vi "AR Drone - Gamepad NavData Video.vi"() -> ()   [LabVIEW 2015]
doc: "Example demonstrating how to control the AR Drone with a joystick or gamepad and simultaneously receive navigation and video data."
uses:
  <vilib>/LVH/AR Drone Toolkit/Decode NavData/Typedefs/NavData Demo.ctl
  <vilib>/LVH/AR Drone Toolkit/Type Defs/Flight Animations.ctl
  <vilib>/Utility/inputDevices.llb/closeJoystick.vi
  <vilib>/LVH/AR Drone Toolkit/AR Drone.lvlib
panel:
  out "Pitching speed":dbl
  out "Hover?":bool
  out "Yawing speed":sgl
  out "Vertical speed":sgl
  in  "Autopilot":bool
  in  "Stop FSM":bool
  in  "Reset":bool
  in  "Start":bool
  in  "Desired yaw":i16
  in  "Restart":bool
  in  "State":i8=1 min=1 max=33 step=1
  out "Downward loop":i8
  out "Snake loop":i8
  out "Upward loop":i8
  out "Current yaw":sgl
  out "Height":i16
  in  "Yaw speed":sgl(slide) min=-1 max=1 scale=-1.0..1.0
  in  "V speed":sgl(slide) min=-1 max=1 scale=-1.0..1.0
  in  "Pitch":sgl(slide) min=-1 max=1 scale=-1.0..1.0
  in  "Roll":sgl(slide) min=-1 max=1 scale=-1.0..1.0
  in  "display/gamepad":bool
  out "Gamepad Output":T1
  in  "Flight Animations":T2 items=["PHI_M30_DEG", "PHI_30_DEG", "THETA_M30_DEG", "THETA_30_DEG", "THETA_20DEG_YAW_200DEG", "THETA_20DEG_YAW_M2000DEG", "TURNAROUND", "TURNAROUND_GODOWN", "YAW_SHAKE", "YAW_DANCE", "PHI_DANCE", "THETA_DANCE", "VZ_DANCE", "WAVE", "PHI_THETA_MIXED", "DOUBLE_PHI_THETA_MIXED", "FLIP_AHEAD", "FLIP_BEHIND", "FLIP_LEFT", "FLIP_RIGHT", "NB_ANIM_MAYDAY"]
  out "Video Stream":picture
  out "NavData Out":T3
  out "Battery Remaining":dbl(slide) scale=0.0..100.0
  out "Axes Output":T4 {"Vertical Speed" scale=-1.0..1.0; "Yaw Speed" scale=-1.0..1.0; "Pitch" scale=-1.0..1.0; "Roll" scale=-1.0..1.0}
  in  "stop":bool
  # "Xbox Controller:\nLeft stick L/R - Roll\nLeft stick D/U - Pitch\nL/R Triggers - Vertical Speed\nRight stick L/R - Yaw Speed"
  # "Xbox Controller:\nA - take off\nB - emergency\nX - hover\nStart - Stop"
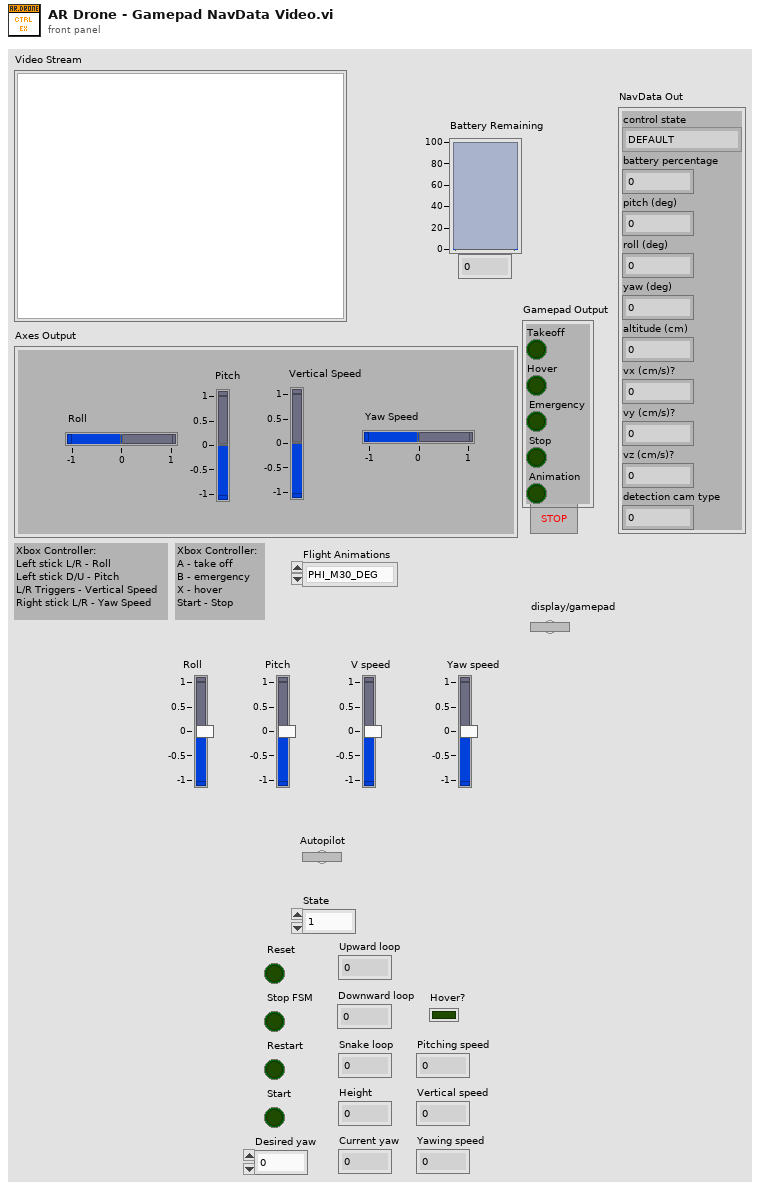
[diagram p1: front panel]
types:
  T1 = cluster{"Takeoff":bool, "Hover":bool, "Emergency":bool, "Stop":bool, "Animation":bool}
  T2 = typedef "AR Drone.lvlib/Flight Animations.ctl" = u16
  T3 = typedef "AR Drone.lvlib/NavData Demo.ctl" = cluster{"control state":enum32{"DEFAULT", "INIT", "LANDING", "FLYING", "HOVERING", "TEST", "TRANS_TAKEOFF", "TRANS_GOTOFIX", "TRANS_LANDING"}, "battery percentage":u32, "pitch (deg)":sgl, "roll (deg)":sgl, "yaw (deg)":sgl, "altitude (cm)":u32, "vx (cm/s)?":sgl, "vy (cm/s)?":sgl, "vz (cm/s)?":sgl, "detection cam type":u32}
  T4 = cluster{"Roll":dbl, "Pitch":dbl, "Vertical Speed":dbl, "Yaw Speed":dbl}
  T5 = typedef "AR Drone.lvlib/AR Drone Resource.ctl" = cluster{"UDP Control Connection":refnum<k16>, "UDP NavData Connection":refnum<k16>, "UDP Video Connection (Drone 1.0)":refnum<k16>, "TCP Video Connection (Drone 2.0)":refnum<k5>, "TCP Control Port Connection":refnum<k5>, "Drone IP address":string, "Drone Command Port":u16, "Drone NavData Port":u16, "Drone Vid Stream Port":u16, "Drone TCP Control Port":u16, "Home IP address":string, "Home Command Port":u16, "Home NavData Port":u16, "Home Vid Stream Port":u16, "Drone Version":i32}
  T6 = cluster{"Roll":sgl, "Pitch":sgl, "V speed":sgl, "Yaw speed":sgl}
  T7 = cluster{"Roll":sgl, "Pitch":sgl, "Vertical Speed":sgl, "Yaw Speed":sgl}
  T8 = cluster{"Yawing speed":sgl, "Pitching speed":dbl, "Vertical speed":sgl, "Yawing speed":sgl}
  T9 = cluster{"Roll":sgl, "Pitching speed":dbl, "V speed":sgl, "Yaw speed":sgl}
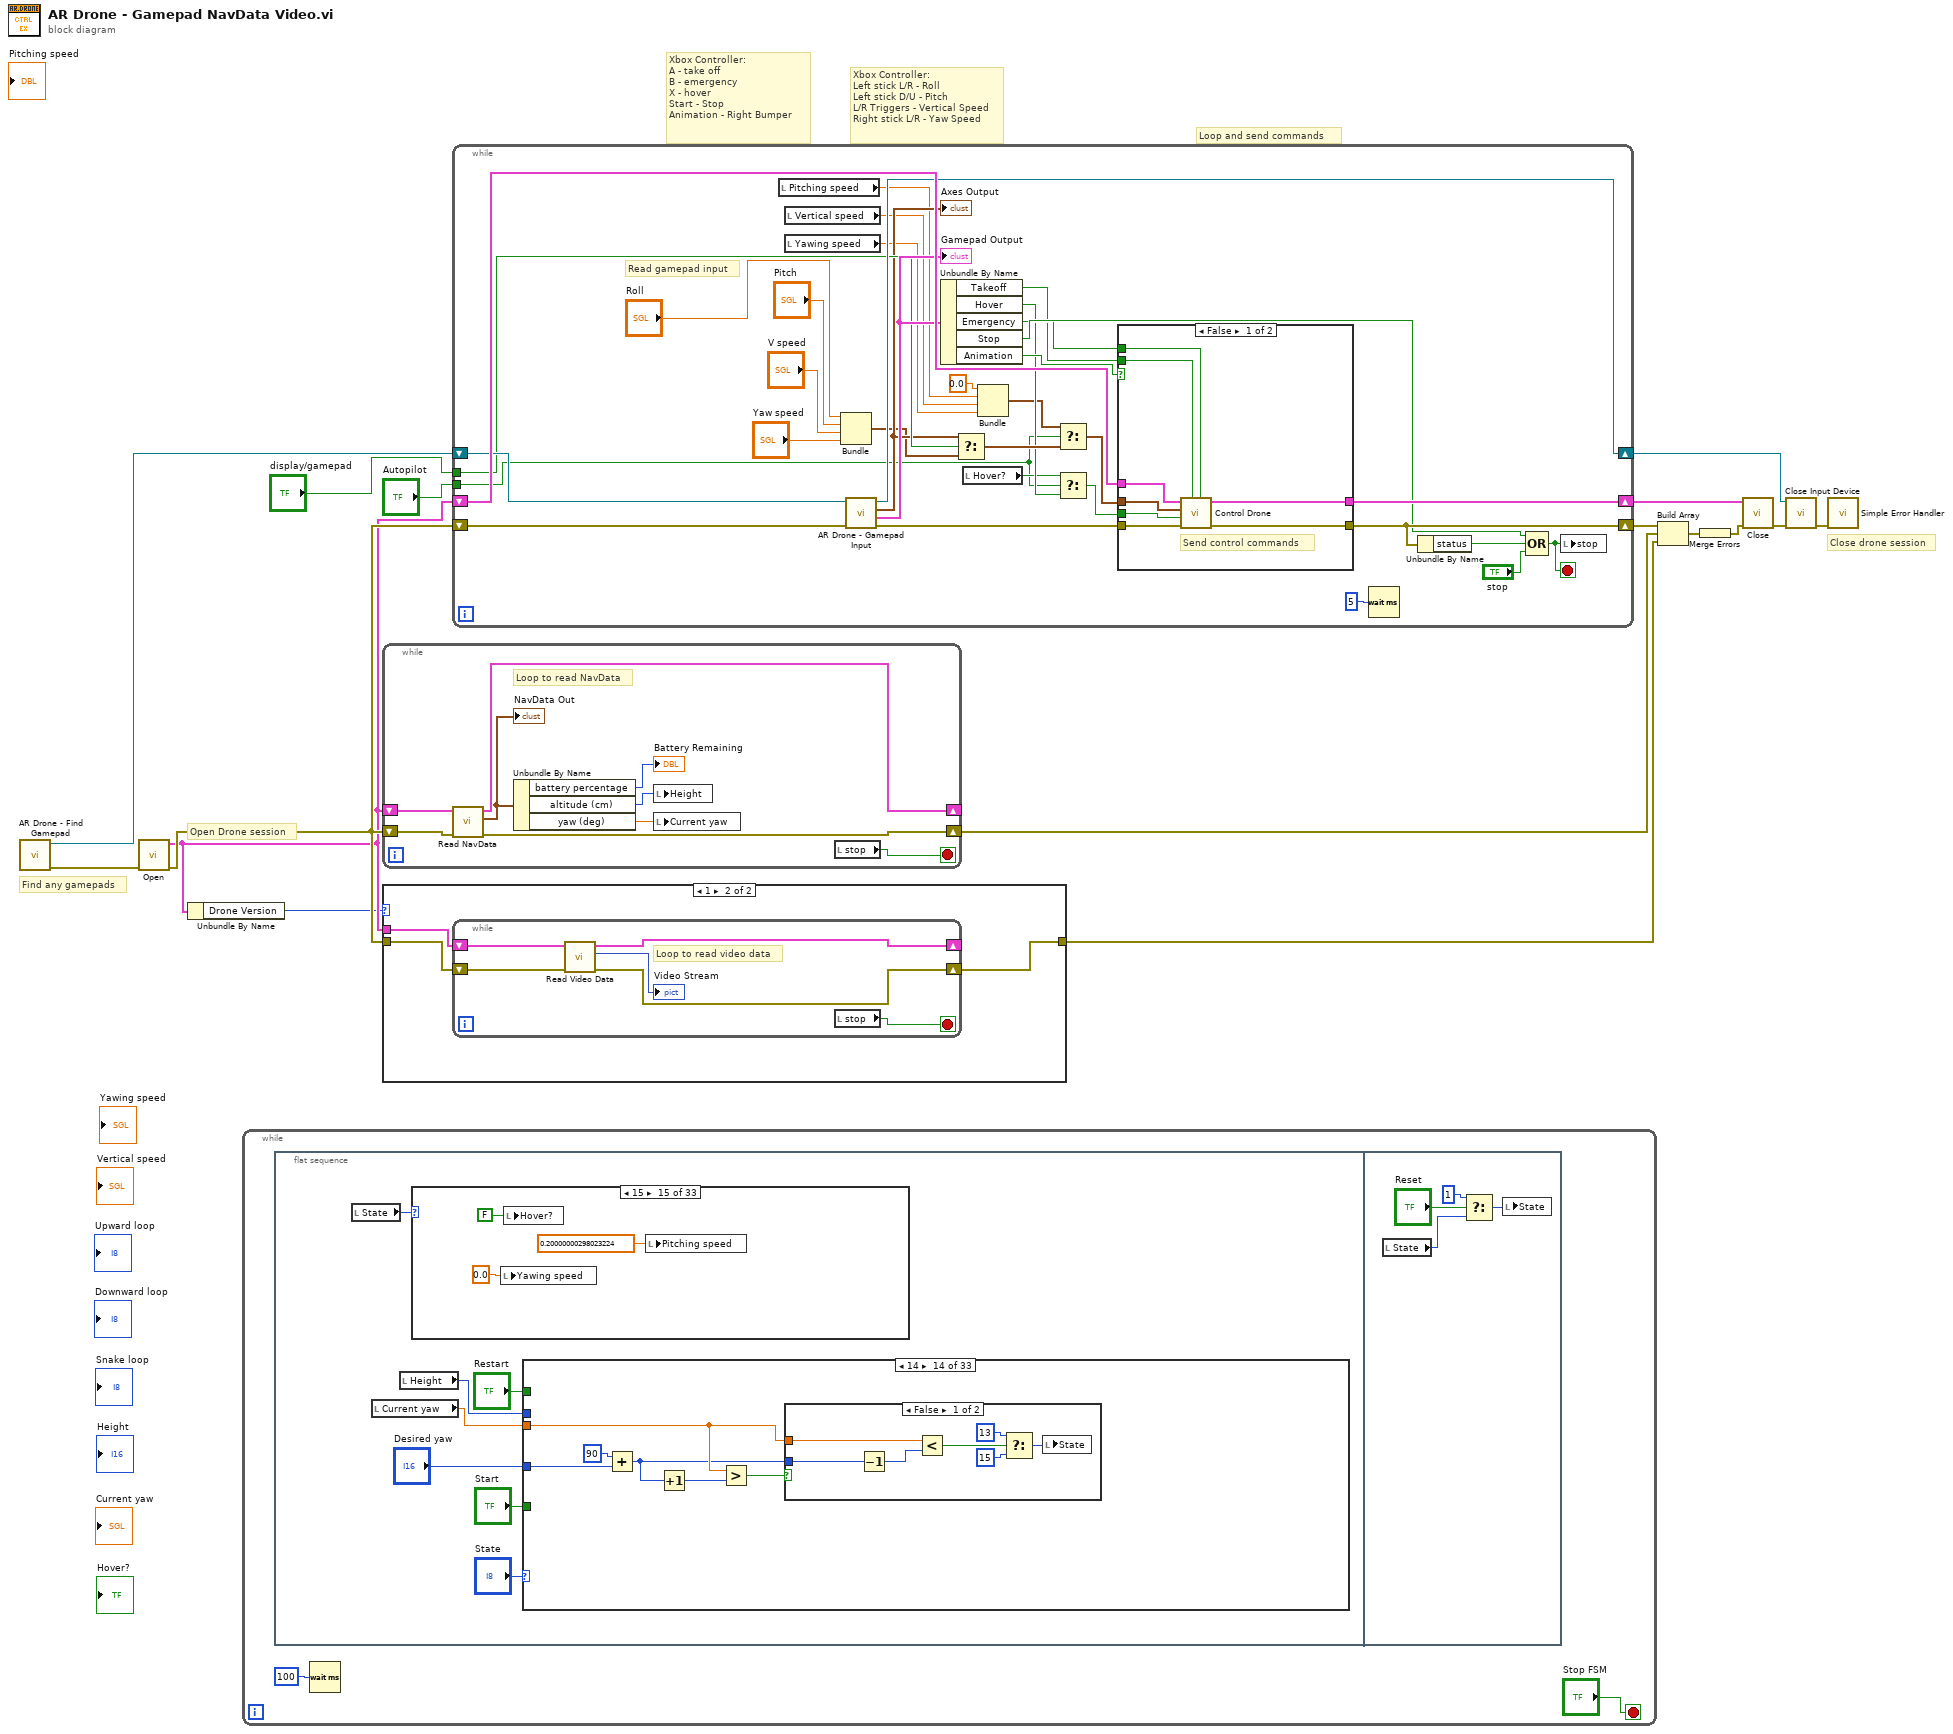
[diagram p0: block diagram]
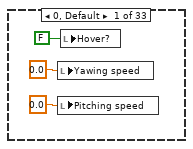
[diagram p2: hidden frame]
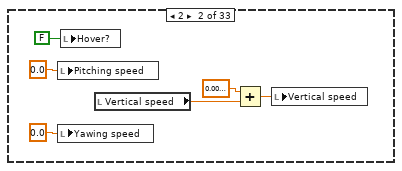
[diagram p3: hidden frame]
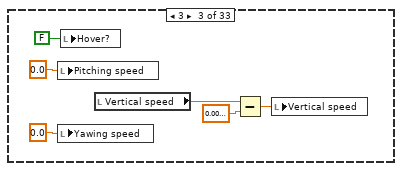
[diagram p4: hidden frame]
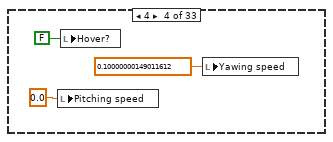
[diagram p5: hidden frame]
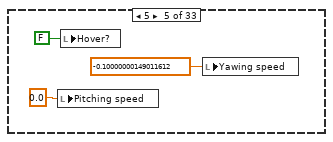
[diagram p6: hidden frame]
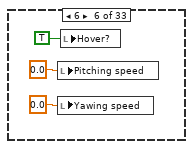
[diagram p7: hidden frame]
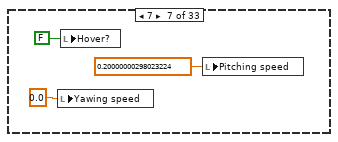
[diagram p8: hidden frame]
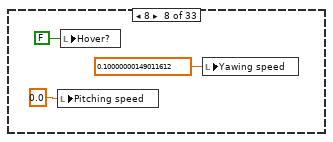
[diagram p9: hidden frame]
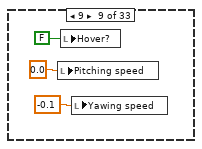
[diagram p10: hidden frame]
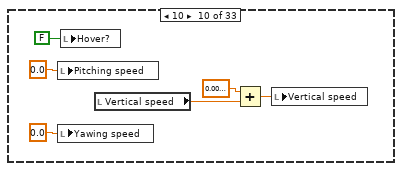
[diagram p11: hidden frame]
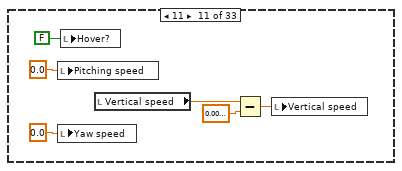
[diagram p12: hidden frame]
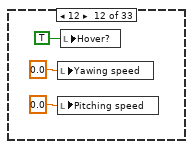
[diagram p13: hidden frame]
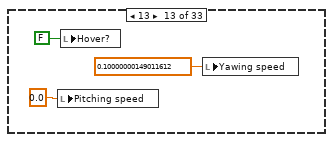
[diagram p14: hidden frame]
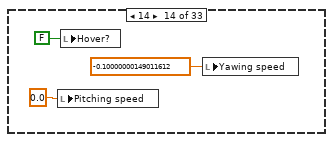
[diagram p15: hidden frame]
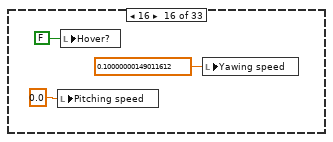
[diagram p16: hidden frame]
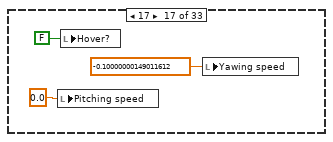
[diagram p17: hidden frame]
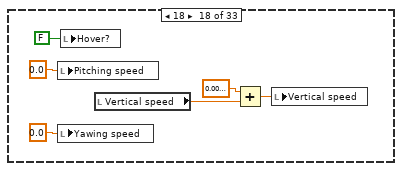
[diagram p18: hidden frame]
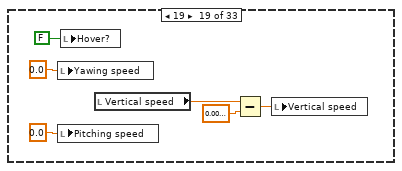
[diagram p19: hidden frame]
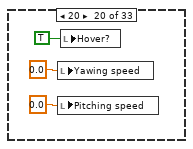
[diagram p20: hidden frame]
diagram:
  # "Loop and send commands"
  # "Close drone session"
  # "Open Drone session"
  # "Find any gamepads"
  # "Xbox Controller:\nLeft stick L/R - Roll\nLeft stick D/U - Pitch\nL/R Triggers - Vertical Speed\nRight stick L/R - Yaw Speed"
  # "Xbox Controller:\nA - take off\nB - emergency\nX - hover\nStart - Stop\nAnimation - Right Bumper"
  n1 = call "AR Drone - Find Gamepad.vi"() -> ("error out"=w11:errorcluster, "Refnum out"=w12:refnum<k1>)  [unwired: 10 in]
  n2 = call <vilib>:"Open.vi"("error in (no error)"=w11) -> ("error out"=w6:errorcluster, "AR Drone Resource"=w4:T5)  [unwired: 9 in]
  n3 = Unbundle By Name(w4) -> ("Drone Version"=w3:i32)
  n4 = while {
    stop <- "Stop FSM" stop-if-true
    n5 = flat-sequence {
      frame #0 {
        n6 = local read "State"() -> (w20:i8)
        n7 = local read "Current yaw"() -> (w23:sgl)
        n8 = local read "Height"() -> (w24:i16)
        n9 = case shown="15" w20 {
          frame 0, Default {
            n10 = local write "Yawing speed"(sgl 0.0 ("Yawing speed")) -> ()
            n11 = local write "Pitching speed"(sgl 0.0 ("Yawing speed")) -> ()
            n12 = local write "Hover?"(FALSE) -> ()
          }
          frame 2 {
            n13 = local write "Pitching speed"(sgl 0.0 ("Yawing speed")) -> ()
            n14 = local write "Yawing speed"(sgl 0.0 ("Yawing speed")) -> ()
            n15 = local write "Hover?"(FALSE) -> ()
            n16 = local read "Vertical speed"() -> (w33:sgl)
            n17 = Add(x=sgl 0.01, y=w33) -> (x+y=w34:sgl)
            n18 = local write "Vertical speed"(w34) -> ()
          }
          frame 3 {
            n19 = local write "Pitching speed"(sgl 0.0 ("Yawing speed")) -> ()
            n20 = local write "Yawing speed"(sgl 0.0 ("Yawing speed")) -> ()
            n21 = local write "Hover?"(FALSE) -> ()
            n22 = local read "Vertical speed"() -> (w39:sgl)
            n23 = Subtract(x=w39, y=sgl 0.01 ("x")) -> (x-y=w40:sgl)
            n24 = local write "Vertical speed"(w40) -> ()
          }
          frame 4 {
            n25 = local write "Pitching speed"(sgl 0.0 ("Yawing speed")) -> ()
            n26 = local write "Hover?"(FALSE) -> ()
            n27 = local write "Yawing speed"(sgl 0.1 ("Yawing speed")) -> ()
          }
          frame 5 {
            n28 = local write "Pitching speed"(sgl 0.0 ("Yawing speed")) -> ()
            n29 = local write "Hover?"(FALSE) -> ()
            n30 = local write "Yawing speed"(sgl -0.1 ("Yawing speed")) -> ()
          }
          frame 6 {
            n31 = local write "Pitching speed"(sgl 0.0 ("Yawing speed")) -> ()
            n32 = local write "Yawing speed"(sgl 0.0 ("Yawing speed")) -> ()
            n33 = local write "Hover?"(TRUE) -> ()
          }
          frame 7 {
            n34 = local write "Yawing speed"(sgl 0.0 ("Yawing speed")) -> ()
            n35 = local write "Hover?"(FALSE) -> ()
            n36 = local write "Pitching speed"(sgl 0.2 ("Yawing speed")) -> ()
          }
          frame 8 {
            n37 = local write "Pitching speed"(sgl 0.0 ("Yawing speed")) -> ()
            n38 = local write "Hover?"(FALSE) -> ()
            n39 = local write "Yawing speed"(sgl 0.1 ("Yawing speed")) -> ()
          }
          frame 9 {
            n40 = local write "Pitching speed"(sgl 0.0 ("Yawing speed")) -> ()
            n41 = local write "Hover?"(FALSE) -> ()
            n42 = local write "Yawing speed"(-0.1 ("Yawing speed")) -> ()
          }
          frame 10 {
            n43 = local write "Pitching speed"(sgl 0.0 ("Yawing speed")) -> ()
            n44 = local write "Yawing speed"(sgl 0.0 ("Yawing speed")) -> ()
            n45 = local write "Hover?"(FALSE) -> ()
            n46 = local read "Vertical speed"() -> (w64:sgl)
            n47 = Add(x=sgl 0.01, y=w64) -> (x+y=w63:sgl)
            n48 = local write "Vertical speed"(w63) -> ()
          }
          frame 11 {
            n49 = local write "Pitching speed"(sgl 0.0 ("Yawing speed")) -> ()
            n50 = local write "Yaw speed"(sgl 0.0 ("Yawing speed")) -> ()
            n51 = local write "Hover?"(FALSE) -> ()
            n52 = local read "Vertical speed"() -> (w69:sgl)
            n53 = Subtract(x=w69, y=sgl 0.01) -> (x-y=w70:sgl)
            n54 = local write "Vertical speed"(w70) -> ()
          }
          frame 12 {
            n55 = local write "Yawing speed"(sgl 0.0 ("Yawing speed")) -> ()
            n56 = local write "Pitching speed"(sgl 0.0 ("Yawing speed")) -> ()
            n57 = local write "Hover?"(TRUE) -> ()
          }
          frame 13 {
            n58 = local write "Pitching speed"(sgl 0.0 ("Yawing speed")) -> ()
            n59 = local write "Hover?"(FALSE) -> ()
            n60 = local write "Yawing speed"(sgl 0.1 ("Yawing speed")) -> ()
          }
          frame 14 {
            n61 = local write "Pitching speed"(sgl 0.0 ("Yawing speed")) -> ()
            n62 = local write "Hover?"(FALSE) -> ()
            n63 = local write "Yawing speed"(sgl -0.1 ("Yawing speed")) -> ()
          }
          frame 15 {
            n64 = local write "Yawing speed"(sgl 0.0 ("Yawing speed")) -> ()
            n65 = local write "Hover?"(FALSE) -> ()
            n66 = local write "Pitching speed"(sgl 0.2 ("Yawing speed")) -> ()
          }
          frame 16 {
            n67 = local write "Pitching speed"(sgl 0.0 ("Yawing speed")) -> ()
            n68 = local write "Hover?"(FALSE) -> ()
            n69 = local write "Yawing speed"(sgl 0.1 ("Yawing speed")) -> ()
          }
          frame 17 {
            n70 = local write "Pitching speed"(sgl 0.0 ("Yawing speed")) -> ()
            n71 = local write "Hover?"(FALSE) -> ()
            n72 = local write "Yawing speed"(sgl -0.1 ("Yawing speed")) -> ()
          }
          frame 18 {
            n73 = local write "Pitching speed"(sgl 0.0 ("Yawing speed")) -> ()
            n74 = local write "Yawing speed"(sgl 0.0 ("Yawing speed")) -> ()
            n75 = local write "Hover?"(FALSE) -> ()
            n76 = local read "Vertical speed"() -> (w94:sgl)
            n77 = Add(x=sgl 0.01, y=w94) -> (x+y=w93:sgl)
            n78 = local write "Vertical speed"(w93) -> ()
          }
          frame 19 {
            n79 = local write "Yawing speed"(sgl 0.0 ("Yawing speed")) -> ()
            n80 = local write "Pitching speed"(sgl 0.0 ("Yawing speed")) -> ()
            n81 = local write "Hover?"(FALSE) -> ()
            n82 = local read "Vertical speed"() -> (w99:sgl)
            n83 = Subtract(x=w99, y=sgl 0.01) -> (x-y=w100:sgl)
            n84 = local write "Vertical speed"(w100) -> ()
          }
          frame 20 {
            n85 = local write "Yawing speed"(sgl 0.0 ("Yawing speed")) -> ()
            n86 = local write "Pitching speed"(sgl 0.0 ("Yawing speed")) -> ()
            n87 = local write "Hover?"(TRUE) -> ()
          }
          frame 21 {
            n88 = local write "Yawing speed"(sgl 0.0 ("Yawing speed")) -> ()
            n89 = local write "Pitching speed"(sgl 0.0 ("Yawing speed")) -> ()
            n90 = local write "Hover?"(FALSE) -> ()
          }
          frame 22 {
            n91 = local write "Pitching speed"(sgl 0.0 ("Yawing speed")) -> ()
            n92 = local write "Hover?"(FALSE) -> ()
            n93 = local write "Yawing speed"(sgl 0.1 ("Yawing speed")) -> ()
          }
          frame 23 {
            n94 = local write "Pitching speed"(sgl 0.0 ("Yawing speed")) -> ()
            n95 = local write "Hover?"(FALSE) -> ()
            n96 = local write "Yawing speed"(sgl -0.1 ("Yawing speed")) -> ()
          }
          frame 24 {
            n97 = local write "Yawing speed"(sgl 0.0 ("Yawing speed")) -> ()
            n98 = local write "Pitching speed"(sgl 0.0 ("Yawing speed")) -> ()
            n99 = local write "Hover?"(FALSE) -> ()
            n100 = local read "Vertical speed"() -> (w118:sgl)
            n101 = Add(x=sgl 0.01, y=w118) -> (x+y=w117:sgl)
            n102 = local write "Vertical speed"(w117) -> ()
          }
          frame 25 {
            n103 = local write "Pitching speed"(sgl 0.0 ("Yawing speed")) -> ()
            n104 = local write "Yawing speed"(sgl 0.0 ("Yawing speed")) -> ()
            n105 = local write "Hover?"(FALSE) -> ()
            n106 = local read "Vertical speed"() -> (w123:sgl)
            n107 = Subtract(x=w123, y=sgl 0.01) -> (x-y=w124:sgl)
            n108 = local write "Vertical speed"(w124) -> ()
          }
          frame 26 {
            n109 = local write "Yawing speed"(sgl 0.0 ("Yawing speed")) -> ()
            n110 = local write "Pitching speed"(sgl 0.0 ("Yawing speed")) -> ()
            n111 = local write "Hover?"(TRUE) -> ()
          }
          frame 27 {
            n112 = local write "Pitching speed"(sgl 0.0 ("Yawing speed")) -> ()
            n113 = local write "Hover?"(FALSE) -> ()
            n114 = local write "Yawing speed"(sgl 0.1 ("Yawing speed")) -> ()
          }
          frame 28 {
            n115 = local write "Pitching speed"(sgl 0.0 ("Yawing speed")) -> ()
            n116 = local write "Hover?"(FALSE) -> ()
            n117 = local write "Yawing speed"(sgl -0.1 ("Yawing speed")) -> ()
          }
          frame 29 {
            n118 = local write "Yawing speed"(sgl 0.0 ("Yawing speed")) -> ()
            n119 = local write "Hover?"(FALSE) -> ()
            n120 = local write "Pitching speed"(sgl 0.2 ("Yawing speed")) -> ()
          }
          frame 30 {
            n121 = local write "Pitching speed"(sgl 0.0 ("Yawing speed")) -> ()
            n122 = local write "Hover?"(FALSE) -> ()
            n123 = local write "Yawing speed"(sgl 0.1 ("Yawing speed")) -> ()
          }
          frame 31 {
            n124 = local write "Pitching speed"(sgl 0.0 ("Yawing speed")) -> ()
            n125 = local write "Hover?"(FALSE) -> ()
            n126 = local write "Yawing speed"(sgl -0.1 ("Yawing speed")) -> ()
          }
          frame 32 {
            n127 = local write "Yawing speed"(sgl 0.0 ("Yawing speed")) -> ()
            n128 = local write "Pitching speed"(sgl 0.0 ("Yawing speed")) -> ()
            n129 = local write "Hover?"(TRUE) -> ()
          }
          frame 33 {
            n130 = local write "Yawing speed"(sgl 0.0 ("Yawing speed")) -> ()
            n131 = local write "Pitching speed"(sgl 0.0 ("Yawing speed")) -> ()
            n132 = local write "Hover?"(FALSE) -> ()
          }
        }
        n133 = case shown="14" "State" {
          tunnel: "Start" -> [w152 _ _ _ _ _ _ _ _ _ _ _ _ _ _ _ _ _ _ _ _ _ _ _ _ _ _ _ _ _ _ _ _]
          tunnel: w24 -> [_ w156 w166 _ _ _ _ _ _ w226 w236 _ _ _ _ _ _ w309 w319 _ _ _ _ w359 w369 _ _ _ _ _ _ _ _]
          tunnel: w23 -> [_ _ _ w178 w189 _ _ w203 w215 _ _ _ w255 w269 _ w281 w295 _ _ _ _ w331 w345 _ _ _ w385 w399 _ w415 w429 _ _]
          tunnel: "Desired yaw" -> [_ _ _ w176 w188 _ _ w202 w214 _ _ _ w252 w268 _ w282 w296 _ _ _ _ w332 w346 _ _ _ w386 w400 _ w414 w428 _ _]
          tunnel: "Restart" -> [_ _ _ _ _ _ _ _ _ _ _ _ _ _ _ _ _ _ _ _ _ _ _ _ _ _ _ _ _ _ _ _ w453]
          frame Default {
            n134 = Select(t=i8 2, s=w152, f=i8 1) -> (s? t:f=w155:i8)
            n135 = local write "Upward loop"(i8 5 ("pic loop")) -> ()
            n136 = local write "Downward loop"(i8 5 ("pic loop 2")) -> ()
            n137 = local write "Snake loop"(i8 3 ("snake loop")) -> ()
            n138 = local write "State"(w155) -> ()
          }
          frame 2 {
            n139 = Greater?(x=w156, y=i16 152) -> (0:w157:bool)
            n140 = case shown="False" w157 {
              tunnel: w156 -> [w164 _]
              frame False {
                n141 = Less?(x=w164, y=i16 148) -> (x < y?=w162:bool)
                n142 = Select(t=i8 2, s=w162, f=i8 4) -> (s? t:f=w159:i8)
                n143 = local write "State"(w159) -> ()
              }
              frame True {
                n144 = local write "State"(i8 3 ("state")) -> ()
              }
            }
          }
          frame 3 {
            n145 = Greater?(x=w166, y=i16 152) -> (0:w168:bool)
            n146 = case shown="True" w168 {
              tunnel: w166 -> [w174 _]
              frame False {
                n147 = Less?(x=w174, y=i16 148) -> (x < y?=w172:bool)
                n148 = Select(t=i8 2, s=w172, f=i8 4) -> (s? t:f=w169:i8)
                n149 = local write "State"(w169) -> ()
              }
              frame True {
                n150 = local write "State"(i8 3 ("state")) -> ()
              }
            }
          }
          frame 4 {
            n151 = Increment(x=w176) -> (x+1=w177:i16)
            n152 = Greater?(x=w178, y=w177) -> (0:w179:bool)
            n153 = case shown="True" w179 {
              tunnel: w178 -> [w186 _]
              tunnel: w176 -> [w180 _]
              frame False {
                n154 = Decrement(x=w180) -> (x-1=w181:i16)
                n155 = Less?(x=w186, y=w181) -> (x < y?=w185:bool)
                n156 = Select(t=i8 4, s=w185, f=i8 6) -> (s? t:f=w182:i8)
                n157 = local write "State"(w182) -> ()
              }
              frame True {
                n158 = local write "State"(i8 5 ("state")) -> ()
              }
            }
          }
          frame 5 {
            n159 = Increment(x=w188) -> (x+1=w191:i16)
            n160 = Greater?(x=w189, y=w191) -> (0:w190:bool)
            n161 = case shown="False" w190 {
              tunnel: w189 -> [w198 _]
              tunnel: w188 -> [w192 _]
              frame False {
                n162 = Decrement(x=w192) -> (x-1=w193:i16)
                n163 = Less?(x=w198, y=w193) -> (x < y?=w197:bool)
                n164 = Select(t=i8 4, s=w197, f=i8 6) -> (s? t:f=w194:i8)
                n165 = local write "State"(w194) -> ()
              }
              frame True {
                n166 = local write "State"(i8 5 ("state")) -> ()
              }
            }
          }
          frame 6 {
            n167 = flat-sequence {
              frame #0 {
                n168 = call "Time Delay"() -> ()  [unwired: 11 in, 1 out]
              }
              frame #1 {
                n169 = local write "State"(i8 7 ("state")) -> ()
              }
            }
          }
          frame 7 {
            n170 = flat-sequence {
              frame #0 {
                n171 = call "Time Delay2"() -> ()  [unwired: 11 in, 1 out]
              }
              frame #1 {
                n172 = local write "State"(i8 8 ("state")) -> ()
              }
            }
          }
          frame 8 {
            n173 = Increment(x=w202) -> (x+1=w204:i16)
            n174 = Greater?(x=w203, y=w204) -> (0:w205:bool)
            n175 = case shown="False" w205 {
              tunnel: w203 -> [w212 _]
              tunnel: w202 -> [w206 _]
              frame False {
                n176 = Decrement(x=w206) -> (x-1=w207:i16)
                n177 = Less?(x=w212, y=w207) -> (x < y?=w211:bool)
                n178 = Select(t=i8 8, s=w211, f=i8 10) -> (s? t:f=w208:i8)
                n179 = local write "State"(w208) -> ()
              }
              frame True {
                n180 = local write "State"(i8 9 ("state")) -> ()
              }
            }
          }
          frame 9 {
            n181 = Increment(x=w214) -> (x+1=w217:i16)
            n182 = Greater?(x=w215, y=w217) -> (0:w216:bool)
            n183 = case shown="True" w216 {
              tunnel: w215 -> [w224 _]
              tunnel: w214 -> [w218 _]
              frame False {
                n184 = Decrement(x=w218) -> (x-1=w219:i16)
                n185 = Less?(x=w224, y=w219) -> (x < y?=w223:bool)
                n186 = Select(t=i8 8, s=w223, f=i8 10) -> (s? t:f=w220:i8)
                n187 = local write "State"(w220) -> ()
              }
              frame True {
                n188 = local write "State"(i8 9 ("state")) -> ()
              }
            }
          }
          frame 10 {
            n189 = Greater?(x=w226, y=i16 152) -> (0:w227:bool)
            n190 = case shown="False" w227 {
              tunnel: w226 -> [w234 _]
              frame False {
                n191 = Less?(x=w234, y=i16 148) -> (x < y?=w232:bool)
                n192 = Select(t=i8 10, s=w232, f=i8 12) -> (s? t:f=w229:i8)
                n193 = local write "State"(w229) -> ()
              }
              frame True {
                n194 = local write "State"(i8 11 ("state")) -> ()
              }
            }
          }
          frame 11 {
            n195 = Greater?(x=w236, y=i16 152) -> (0:w238:bool)
            n196 = case shown="False" w238 {
              tunnel: w236 -> [w244 _]
              frame False {
                n197 = Less?(x=w244, y=i16 148) -> (x < y?=w242:bool)
                n198 = Select(t=i8 10, s=w242, f=i8 12) -> (s? t:f=w239:i8)
                n199 = local write "State"(w239) -> ()
              }
              frame True {
                n200 = local write "State"(i8 11 ("state")) -> ()
              }
            }
          }
          frame 12 {
            n201 = flat-sequence {
              frame #0 {
                n202 = call "Time Delay3"() -> ()  [unwired: 11 in, 1 out]
              }
              frame #1 {
                n203 = local read "Upward loop"() -> (w250:i8)
                n204 = Decrement(x=w250) -> (x-1=w251:i8)
                n205 = local write "Upward loop"(w251) -> ()
                n206 = Equal To 0?(x=w251) -> (x = 0?=w246:bool)
                n207 = Select(t=i8 13, s=w246, f=i8 7) -> (s? t:f=w249:i8)
                n208 = local write "State"(w249) -> ()
              }
            }
          }
          frame 13 {
            n209 = Add(x=i16 90, y=w252) -> (x+y=w253:i16)
            n210 = Increment(x=w253) -> (x+1=w257:i16)
            n211 = Greater?(x=w255, y=w257) -> (0:w256:bool)
            n212 = case shown="True" w256 {
              tunnel: w255 -> [w264 _]
              tunnel: w253 -> [w258 _]
              frame False {
                n213 = Decrement(x=w258) -> (x-1=w259:i16)
                n214 = Less?(x=w264, y=w259) -> (x < y?=w263:bool)
                n215 = Select(t=i8 13, s=w263, f=i8 15) -> (s? t:f=w260:i8)
                n216 = local write "State"(w260) -> ()
              }
              frame True {
                n217 = local write "State"(i8 14 ("state")) -> ()
              }
            }
          }
          frame 14 {
            n218 = Add(x=i16 90, y=w268) -> (x+y=w267:i16)
            n219 = Increment(x=w267) -> (x+1=w270:i16)
            n220 = Greater?(x=w269, y=w270) -> (0:w271:bool)
            n221 = case shown="False" w271 {
              tunnel: w269 -> [w278 _]
              tunnel: w267 -> [w272 _]
              frame False {
                n222 = Decrement(x=w272) -> (x-1=w273:i16)
                n223 = Less?(x=w278, y=w273) -> (x < y?=w277:bool)
                n224 = Select(t=i8 13, s=w277, f=i8 15) -> (s? t:f=w274:i8)
                n225 = local write "State"(w274) -> ()
              }
              frame True {
                n226 = local write "State"(i8 14 ("state")) -> ()
              }
            }
          }
          frame 15 {
            n227 = flat-sequence {
              frame #0 {
                n228 = call "Time Delay4"() -> ()  [unwired: 11 in, 1 out]
              }
              frame #1 {
                n229 = local write "State"(i8 16 ("state")) -> ()
              }
            }
          }
          frame 16 {
            n230 = Add(x=i16 180, y=w282) -> (x+y=w286:i16)
            n231 = Increment(x=w286) -> (x+1=w283:i16)
            n232 = Greater?(x=w281, y=w283) -> (0:w284:bool)
            n233 = case shown="True" w284 {
              tunnel: w281 -> [w293 _]
              tunnel: w286 -> [w287 _]
              frame False {
                n234 = Decrement(x=w287) -> (x-1=w288:i16)
                n235 = Less?(x=w293, y=w288) -> (x < y?=w292:bool)
                n236 = Select(t=i8 16, s=w292, f=i8 18) -> (s? t:f=w289:i8)
                n237 = local write "State"(w289) -> ()
              }
              frame True {
                n238 = local write "State"(i8 17 ("state")) -> ()
              }
            }
          }
          frame 17 {
            n239 = Add(x=i16 180, y=w296) -> (x+y=w300:i16)
            n240 = Increment(x=w300) -> (x+1=w297:i16)
            n241 = Greater?(x=w295, y=w297) -> (0:w298:bool)
            n242 = case shown="True" w298 {
              tunnel: w295 -> [w307 _]
              tunnel: w300 -> [w301 _]
              frame False {
                n243 = Decrement(x=w301) -> (x-1=w302:i16)
                n244 = Less?(x=w307, y=w302) -> (x < y?=w306:bool)
                n245 = Select(t=i8 16, s=w306, f=i8 18) -> (s? t:f=w303:i8)
                n246 = local write "State"(w303) -> ()
              }
              frame True {
                n247 = local write "State"(i8 17 ("state")) -> ()
              }
            }
          }
          frame 18 {
            n248 = Greater?(x=w309, y=i16 152) -> (0:w311:bool)
            n249 = case shown="True" w311 {
              tunnel: w309 -> [w317 _]
              frame False {
                n250 = Less?(x=w317, y=i16 148) -> (x < y?=w315:bool)
                n251 = Select(t=i8 18, s=w315, f=i8 20) -> (s? t:f=w312:i8)
                n252 = local write "State"(w312) -> ()
              }
              frame True {
                n253 = local write "State"(i8 19 ("state")) -> ()
              }
            }
          }
          frame 19 {
            n254 = Greater?(x=w319, y=i16 152) -> (0:w321:bool)
            n255 = case shown="True" w321 {
              tunnel: w319 -> [w327 _]
              frame False {
                n256 = Less?(x=w327, y=i16 148) -> (x < y?=w325:bool)
                n257 = Select(t=i8 18, s=w325, f=i8 20) -> (s? t:f=w322:i8)
                n258 = local write "State"(w322) -> ()
              }
              frame True {
                n259 = local write "State"(i8 19 ("state")) -> ()
              }
            }
          }
          frame 20 {
            n260 = flat-sequence {
              frame #0 {
                n261 = call "Time Delay5"() -> ()  [unwired: 11 in, 1 out]
              }
              frame #1 {
                n262 = local write "State"(i8 21 ("state")) -> ()
              }
            }
          }
          frame 21 {
            n263 = flat-sequence {
              frame #0 {
                n264 = call "Time Delay6"() -> ()  [unwired: 11 in, 1 out]
              }
              frame #1 {
                n265 = local write "State"(i8 22 ("state")) -> ()
              }
            }
          }
          frame 22 {
            n266 = Add(x=i16 180, y=w332) -> (x+y=w333:i16)
            n267 = Increment(x=w333) -> (x+1=w336:i16)
            n268 = Greater?(x=w331, y=w336) -> (0:w335:bool)
            n269 = case shown="True" w335 {
              tunnel: w331 -> [w343 _]
              tunnel: w333 -> [w337 _]
              frame False {
                n270 = Decrement(x=w337) -> (x-1=w338:i16)
                n271 = Less?(x=w343, y=w338) -> (x < y?=w342:bool)
                n272 = Select(t=i8 22, s=w342, f=i8 24) -> (s? t:f=w339:i8)
                n273 = local write "State"(w339) -> ()
              }
              frame True {
                n274 = local write "State"(i8 23 ("state")) -> ()
              }
            }
          }
          frame 23 {
            n275 = Add(x=i16 180, y=w346) -> (x+y=w347:i16)
            n276 = Increment(x=w347) -> (x+1=w350:i16)
            n277 = Greater?(x=w345, y=w350) -> (0:w349:bool)
            n278 = case shown="True" w349 {
              tunnel: w345 -> [w357 _]
              tunnel: w347 -> [w351 _]
              frame False {
                n279 = Decrement(x=w351) -> (x-1=w352:i16)
                n280 = Less?(x=w357, y=w352) -> (x < y?=w356:bool)
                n281 = Select(t=i8 22, s=w356, f=i8 24) -> (s? t:f=w353:i8)
                n282 = local write "State"(w353) -> ()
              }
              frame True {
                n283 = local write "State"(i8 23 ("state")) -> ()
              }
            }
          }
          frame 24 {
            n284 = Greater?(x=w359, y=i16 152) -> (0:w360:bool)
            n285 = case shown="True" w360 {
              tunnel: w359 -> [w367 _]
              frame False {
                n286 = Less?(x=w367, y=i16 148) -> (x < y?=w365:bool)
                n287 = Select(t=i8 24, s=w365, f=i8 26) -> (s? t:f=w362:i8)
                n288 = local write "State"(w362) -> ()
              }
              frame True {
                n289 = local write "State"(i8 25 ("state")) -> ()
              }
            }
          }
          frame 25 {
            n290 = Greater?(x=w369, y=i16 152) -> (0:w370:bool)
            n291 = case shown="True" w370 {
              tunnel: w369 -> [w377 _]
              frame False {
                n292 = Less?(x=w377, y=i16 148) -> (x < y?=w375:bool)
                n293 = Select(t=i8 24, s=w375, f=i8 26) -> (s? t:f=w372:i8)
                n294 = local write "State"(w372) -> ()
              }
              frame True {
                n295 = local write "State"(i8 25 ("state")) -> ()
              }
            }
          }
          frame 26 {
            n296 = flat-sequence {
              frame #0 {
                n297 = call "Time Delay7"() -> ()  [unwired: 11 in, 1 out]
              }
              frame #1 {
                n298 = local read "Downward loop"() -> (w383:i8)
                n299 = Decrement(x=w383) -> (x-1=w384:i8)
                n300 = local write "Downward loop"(w384) -> ()
                n301 = Equal To 0?(x=w384) -> (x = 0?=w379:bool)
                n302 = Select(t=i8 27, s=w379, f=i8 21) -> (s? t:f=w382:i8)
                n303 = local write "State"(w382) -> ()
              }
            }
          }
          frame 27 {
            n304 = Add(x=i16 90, y=w386) -> (x+y=w390:i16)
            n305 = Increment(x=w390) -> (x+1=w387:i16)
            n306 = Greater?(x=w385, y=w387) -> (0:w388:bool)
            n307 = case shown="True" w388 {
              tunnel: w385 -> [w397 _]
              tunnel: w390 -> [w391 _]
              frame False {
                n308 = Decrement(x=w391) -> (x-1=w392:i16)
                n309 = Less?(x=w397, y=w392) -> (x < y?=w396:bool)
                n310 = Select(t=i8 27, s=w396, f=i8 29) -> (s? t:f=w393:i8)
                n311 = local write "State"(w393) -> ()
              }
              frame True {
                n312 = local write "State"(i8 28 ("state")) -> ()
              }
            }
          }
          frame 28 {
            n313 = Add(x=i16 90, y=w400) -> (x+y=w401:i16)
            n314 = Increment(x=w401) -> (x+1=w404:i16)
            n315 = Greater?(x=w399, y=w404) -> (0:w403:bool)
            n316 = case shown="False" w403 {
              tunnel: w399 -> [w411 _]
              tunnel: w401 -> [w405 _]
              frame False {
                n317 = Decrement(x=w405) -> (x-1=w406:i16)
                n318 = Less?(x=w411, y=w406) -> (x < y?=w410:bool)
                n319 = Select(t=i8 27, s=w410, f=i8 29) -> (s? t:f=w407:i8)
                n320 = local write "State"(w407) -> ()
              }
              frame True {
                n321 = local write "State"(i8 28 ("state")) -> ()
              }
            }
          }
          frame 29 {
            n322 = flat-sequence {
              frame #0 {
                n323 = call "Time Delay8"() -> ()  [unwired: 11 in, 1 out]
              }
              frame #1 {
                n324 = local write "State"(i8 30 ("state")) -> ()
              }
            }
          }
          frame 30 {
            n325 = Add(x=i16 180, y=w414) -> (x+y=w416:i16)
            n326 = Increment(x=w416) -> (x+1=w419:i16)
            n327 = Greater?(x=w415, y=w419) -> (0:w418:bool)
            n328 = case shown="True" w418 {
              tunnel: w415 -> [w426 _]
              tunnel: w416 -> [w420 _]
              frame False {
                n329 = Decrement(x=w420) -> (x-1=w421:i16)
                n330 = Less?(x=w426, y=w421) -> (x < y?=w425:bool)
                n331 = Select(t=i8 30, s=w425, f=i8 32) -> (s? t:f=w422:i8)
                n332 = local write "State"(w422) -> ()
              }
              frame True {
                n333 = local write "State"(i8 31 ("state")) -> ()
              }
            }
          }
          frame 31 {
            n334 = Add(x=i16 180, y=w428) -> (x+y=w430:i16)
            n335 = Increment(x=w430) -> (x+1=w433:i16)
            n336 = Greater?(x=w429, y=w433) -> (0:w432:bool)
            n337 = case shown="True" w432 {
              tunnel: w429 -> [w440 _]
              tunnel: w430 -> [w434 _]
              frame False {
                n338 = Decrement(x=w434) -> (x-1=w435:i16)
                n339 = Less?(x=w440, y=w435) -> (x < y?=w439:bool)
                n340 = Select(t=i8 30, s=w439, f=i8 32) -> (s? t:f=w436:i8)
                n341 = local write "State"(w436) -> ()
              }
              frame True {
                n342 = local write "State"(i8 31 ("state")) -> ()
              }
            }
          }
          frame 32 {
            n343 = flat-sequence {
              frame #0 {
                n344 = call "Time Delay9"() -> ()  [unwired: 11 in, 1 out]
              }
              frame #1 {
                n345 = local write "Upward loop"(i8 5 ("pic loop 1")) -> ()
                n346 = local write "Downward loop"(i8 5 ("pic loop 2")) -> ()
                n347 = local read "Snake loop"() -> (w446:i8)
                n348 = Decrement(x=w446) -> (x-1=w447:i8)
                n349 = Equal To 0?(x=w447) -> (x = 0?=w442:bool)
                n350 = local write "Snake loop"(w447) -> ()
                n351 = Select(t=i8 33, s=w442, f=i8 7) -> (s? t:f=w445:i8)
                n352 = local write "State"(w445) -> ()
              }
            }
          }
          frame 33 {
            n353 = Select(t=i8 1, s=w453, f=i8 33) -> (s? t:f=w452:i8)
            n354 = local write "State"(w452) -> ()
          }
        }
      }
      frame #1 {
        n355 = local read "State"() -> (w456:i8)
        n356 = Select(t=i8 1, s="Reset", f=w456) -> (s? t:f=w457:i8)
        n357 = local write "State"(w457) -> ()
      }
    }
    n358 = Wait (ms)(milliseconds to wait=u32 100) -> ()  [unwired: 1 out]
  }
  n359 = while {
    shift-right: [w465] -> _
    shift-left: w4 -> [w466]
    shift-right: [w463] -> w8
    shift-left: w6 -> [w464]
    stop <- w461 stop-if-true
    # "Loop to read NavData"
    n360 = call <vilib>:"Read NavData.vi"("error in (no error)"=w464, "AR Drone Resource"=w466) -> ("error out"=w463:errorcluster, "NavData Out"=w460:T3, "AR Drone Resource Out"=w465:T5)  [unwired: 7 in]
    "NavData Out" <- w460
    n361 = Unbundle By Name(w460) -> ("battery percentage"=→"Battery Remaining":u32, "altitude (cm)"=w459:u32, "yaw (deg)"=w458:sgl)
    n362 = local write "Height"(w459) -> ()
    n363 = local write "Current yaw"(w458) -> ()
    n364 = local read "stop"() -> (w461:bool)
  }
  n365 = case shown="1" w3 {
    tunnel: w4 -> [_ w470]
    tunnel: [w467 w469] -> w7
    tunnel: w6 -> [w467 w468]
    frame 2, Default {
      # "If Drone 2.0, no streaming in line"
    }
    frame 1 {
      n366 = while {
        shift-right: [w474] -> _
        shift-left: w470 -> [w476]
        shift-right: [w473] -> w469
        shift-left: w468 -> [w475]
        stop <- w471 stop-if-true
        # "Loop to read video data"
        n367 = call <vilib>:"Read Video Data.vi"("error in (no error)"=w475, "AR Drone Resource"=w476) -> ("error out"=w473:errorcluster, "Video Stream"=→"Video Stream":picture, "AR Drone Resource Out"=w474:T5)  [unwired: 7 in]
        n368 = local read "stop"() -> (w471:bool)
      }
    }
  }
  n369 = while {
    shift-right: [w509] -> w16
    shift-left: w4 -> [w510]
    shift-right: [w508] -> w9
    shift-left: w6 -> [w503]
    shift-right: [w500] -> w15
    shift-left: w12 -> [w504]
    tunnel: "display/gamepad" -> [w494]
    tunnel: "Autopilot" -> [w482]
    stop <- w496 stop-if-true
    # "Read gamepad input"
    n370 = local read "Pitching speed"() -> (w481:dbl)
    n371 = local read "Vertical speed"() -> (w478:sgl)
    n372 = local read "Yawing speed"() -> (w479:sgl)
    n373 = Bundle("Roll"="Roll", "Pitch"="Pitch", "V speed"="V speed", "Yaw speed"="Yaw speed") -> (w489:T6)  [unwired: 1 in]
    n374 = call "AR Drone - Gamepad Input.vi"("error in (no error)"=w503, "Refnum in"=w504) -> ("error out"=w502:errorcluster, "Gamepad Output"=w501:T1, "Control Cluster"=w493:T7, "Refnum out"=w500:refnum<k1>)  [unwired: 6 in]
    "Axes Output" <- w493
    "Gamepad Output" <- w501
    n375 = Unbundle By Name(w501) -> ("Takeoff"=w497:bool, "Hover"=w484:bool, "Emergency"=w498:bool, "Stop"=w499:bool, "Animation"=w495:bool)
    n376 = Select(t=w493, s=w494, f=w489) -> (s? t:f=w487:T6)
    n377 = local read "Hover?"() -> (w483:bool)
    n378 = Bundle("Yawing speed"=sgl 0.0, "Pitching speed"=w481, "Vertical speed"=w478, "Yawing speed"=w479) -> (w477:T8)  [unwired: 1 in]
    n379 = Select(t=w477, s=w482, f=w487) -> (s? t:f=w486:T9)
    n380 = Select(t=w483, s=w482, f=w484) -> (s? t:f=w485:bool)
    n381 = case shown="False" w495 {
      tunnel: w510 -> [w518 w521]
      tunnel: [w517 w519] -> w509
      tunnel: [w516 w520] -> w508
      tunnel: w502 -> [w515 w522]
      tunnel: w486 -> [w514 _]
      tunnel: w498 -> [w513 _]
      tunnel: w485 -> [w512 _]
      tunnel: w497 -> [w511 _]
      frame False {
        # "Send control commands"
        n382 = call <vilib>:"Control Drone.vi"("Emergency Landing"=w513, "Takeoff/Land"=w511, "error in (no error)"=w515, "Hover"=w512, "Control Cluster"=w514, "AR Drone Resource"=w518) -> ("error out"=w516:errorcluster, "AR Drone Resource Out"=w517:T5)  [unwired: 4 in]
      }
      frame True {
        n383 = call <vilib>:"Execute Animation.vi"("error in (no error)"=w522, "Flight Animation"="Flight Animations", "AR Drone Resource"=w521) -> ("error out"=w520:errorcluster, "AR Drone Resource Out"=w519:T5)  [unwired: 7 in]
      }
    }
    n384 = Wait (ms)(milliseconds to wait=u32 5) -> ()  [unwired: 1 out]
    n385 = Unbundle By Name(w508) -> ("status"=w506:bool)
    n386 = Compound Arithmetic op=OR(w499, w506, "stop") -> (w496:bool)
    n387 = local write "stop"(w496) -> ()
  }
  n388 = Build Array(w9, w8, w7) -> (w5:errorcluster[])
  n389 = Merge Errors(w5) -> (w10:errorcluster)
  n390 = call <vilib>:"Close.vi"("error in (no error)"=w10, "AR Drone Resource"=w16) -> ("error out"=w14:errorcluster)  [unwired: 9 in]
  n391 = call-poly <vilib>:"Close Input Device.vi"("error in (no error)"=w14, "device ID"=w15) -> ("error out"=w13:errorcluster)  [unwired: 8 in]
  n392 = call <vilib>:"Simple Error Handler.vi"("error in (no error)"=w13) -> ()  [unwired: 4 in, 5 out]
